vi "测试状态输出.vi"(8 "error in (no error)":errorcluster caption="错误输入（无错误）", 11 "TimingControl输入":refnum<class "TimingControl.lvclass">) -> (0 "error out":errorcluster caption="错误输出", 2 "测试状态":T1, 3 "TimingControl输出":refnum<class "TimingControl.lvclass">)   [LabVIEW 2016, in "TimingControl.lvlib" / "TimingControl.lvclass"]
uses:
  TimingControl.lvclass
  TimingControl.lvclass/TimingControl.ctl
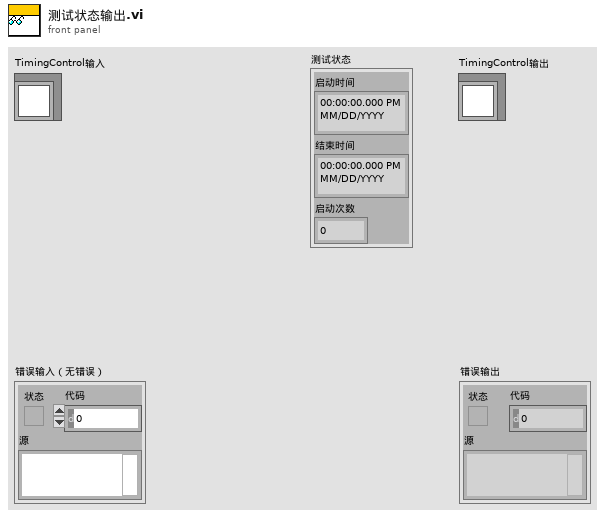
[diagram p1: front panel]
types:
  T1 = cluster{"启动时间":timestamp, "结束时间":timestamp, "启动次数":i32}
  T2 = typedef "TimingControl.lvlib/TimingControl.lvclass/State Data.ctl" = cluster{"仪器时间":timestamp, "仪器运行状态":bool, "配置文件路径":path, "测量参数":T3, "测试状态":cluster{"启动时间":timestamp, "结束时间":timestamp, "启动次数":i32}, "配置信息":T4}
  T3 = typedef "TimingControl.lvlib/TimingControl.lvclass/测量参数.ctl" = cluster{"测量参数":string[]}
  T4 = typedef "TimingControl.lvlib/TimingControl.lvclass/配置信息.ctl" = cluster{"每周启动":T5, "每月启动":T6, "周期模式":T7, "测量参数":T3, "定点周期":T8, "间隔启动":T10, "配置时间":timestamp, "配置":cluster{"测量参数":string, "控制命令":T11, "启动时间":string, "启动次数":u16, "启动间隔":dbl, "每周启动":T5, "每月启动":T6, "每日启动":enum16{"关闭", "每日"}}[]}
  T5 = typedef "TimingControl.lvlib/TimingControl.lvclass/每周启动.ctl" = enum16{"关闭", "周日", "周一", "周二", "周三", "周四", "周五", "周六"}
  T6 = typedef "TimingControl.lvlib/TimingControl.lvclass/每月启动.ctl" = enum16{"关闭", "1号", "2号", "3号", "4号", "5号", "6号", "7号", "8号", "9号", "10号", "11号", "12号", "13号", "14号", "15号", "16号", "17号", "18号", "19号", "20号", "21号", "22号", "23号", "24号", "25号", "26号", "27号", "28号", "29号", "30号", "31号"}
  T7 = typedef "TimingControl.lvlib/TimingControl.lvclass/周期模式设置.ctl" = enum16{"定点模式", "间隔模式"}
  T8 = typedef "TimingControl.lvlib/TimingControl.lvclass/定点周期设置.ctl" = cluster{"时间":u16, "启动命令":T9}
  T9 = typedef "TimingControl.lvlib/TimingControl.lvclass/启动命令选择.ctl" = enum16{"", "水样测试", "标样核查", "零点核查", "跨度核查", "空白测试", "平行样测试", "加标回收", "空白校准", "标样校准", "初始化(清洗)"}
  T10 = typedef "TimingControl.lvlib/TimingControl.lvclass/间隔启动设置.ctl" = cluster{"启动命令":T9, "启动间隔":dbl, "启动次数":i32}
  T11 = typedef "TimingControl.lvlib/TimingControl.lvclass/国标控制命令.ctl" = enum16{"启动测量", "标样核查", "零点核查", "跨度核查", "空白测试", "平行样测试", "加标回收", "空白校准", "标样校准", "初始化（清洗）", "停止测试", "仪器重启", "校时", "模式设置", "测量间隔设置"}
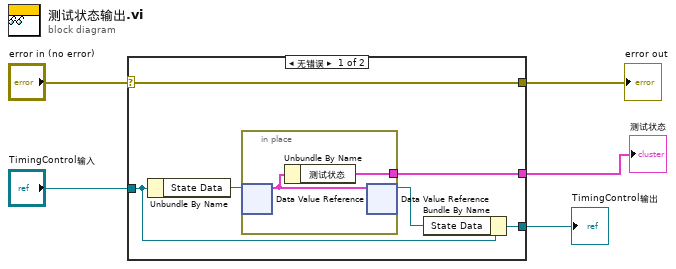
[diagram p0: block diagram]
diagram:
  n1 = case shown="无错误" "error in (no error)" {
    selector: "error in (no error)" -> [w11 w14]
    tunnel: [w11 w14] -> w4
    tunnel: [w6 w15] -> w2
    tunnel: "TimingControl输入" -> [w8 w15]
    tunnel: [w9 _] -> w1
    frame No Error {
      n2 = Unbundle By Name(w8) -> ("State Data"=w10:refnum<data-value>)
      n3 = in-place {
        in-place-border: [w13] -> w9
        n4 = in-place-dvr #1(w10) -> (w12:T2)  [unwired: 1 out]
        n5 = Unbundle By Name(w12) -> ("测试状态"=w13:T1)
        n6 = in-place-dvr #1(w12) -> (w7:refnum<data-value>)  [unwired: 1 out]
      }
      n7 = Bundle By Name(cluster=w8, "State Data"=w7) -> (w6:refnum<class "TimingControl.lvclass">)
    }
    frame Error {
    }
  }
  "error out" <- w4
  "TimingControl输出" <- w2
  "测试状态" <- w1
